vi "PingCore.vi"(8 "error in (no error)":errorcluster, 10 "Timeout (ms)":i32=60000, 11 "MicronGRPCClient in":refnum<class "MicronGRPCClient.lvclass">) -> (0 "error out":errorcluster, 2 "Response":string, 3 "MicronGRPCClient out":refnum<class "MicronGRPCClient.lvclass">)   [LabVIEW 2019, in "MicronGRPCClient.lvclass"]
uses:
  MicronGRPCClient.lvclass
  MicronCLI/Typedefs/Message.ctl
  MicronCLI/Typedefs/ServiceDetails.ctl
  MicronCLI/MicronCLI.lvclass
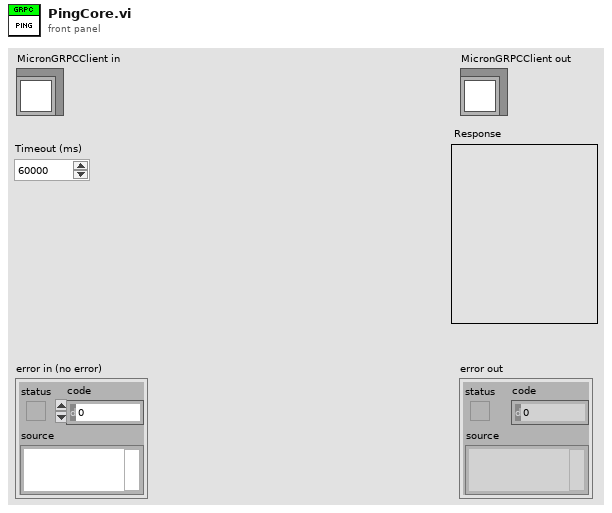
[diagram p1: front panel]
types:
  T1 = typedef "MicronCLI.lvclass/ServiceDetails.ctl" = cluster{"Network":string, "ServiceID":string}
  T2 = typedef "MicronCLI.lvclass/Message.ctl" = cluster{"Command":string, "Payload":string}
  T3 = typedef "MicronClient.lvclass/ServiceDetails.ctl" = cluster{"MicronPath":path, "Network":string, "ServiceID":string, "Port":i32, "FullyQualifiedName":string, "UI":string, "Args":string, "Mode":string, "AutoRestartOnError?":bool, "Simulate?":bool}
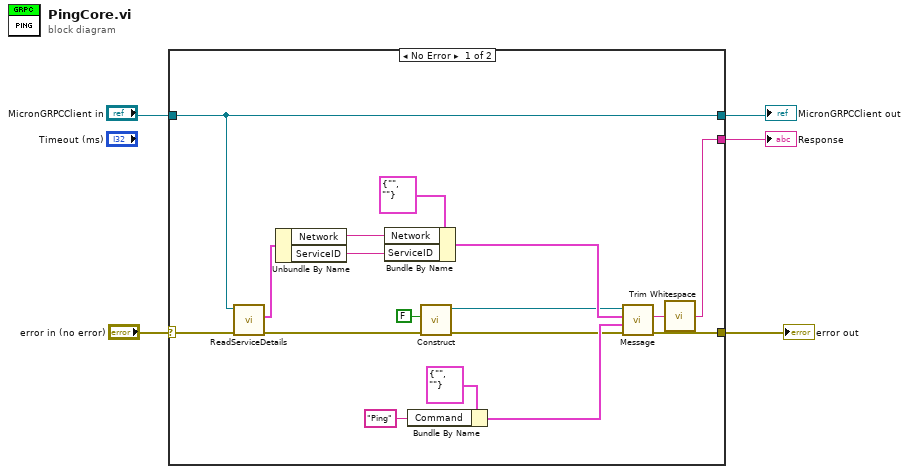
[diagram p0: block diagram]
diagram:
  n1 = case shown="No Error" "error in (no error)" {
    selector: "error in (no error)" -> [w10 w23]
    tunnel: "MicronGRPCClient in" -> [w9 w24]
    tunnel: [w6 _] -> w4
    tunnel: [w11 w23] -> w3
    tunnel: [w9 w24] -> w1
    frame No Error {
      n2 = call-dynamic "ReadServiceDetails.vi"("error in (no error)"=w10, "MicronGRPCClient in"=w9) -> ("error out"=w12:errorcluster, "ServiceDetails"=w18:T3)  [unwired: 7 in, 1 out]
      n3 = Unbundle By Name(w18) -> ("Network"=w16:string, "ServiceID"=w15:string)
      n4 = Bundle By Name(cluster=T1 {"Network"="", "ServiceID"=""} ("Service"), "Network"=w16, "ServiceID"=w15) -> (w14:T1)
      n5 = Bundle By Name(cluster=T2 {"Command"="", "Payload"=""} ("Message"), "Command"="Ping") -> (w19:T2)
      n6 = call "Construct.vi"("error in (no error)"=w12, "SkipIfNotPresent?"=FALSE) -> ("error out"=w7:errorcluster, "MicronCLI out"=w8:refnum<class "MicronCLI.lvclass">)  [unwired: 7 in, 1 out]
      n7 = call-dynamic "Message.vi"("error in (no error)"=w7, "Message"=w19, "Service"=w14, "MicronCLI in"=w8) -> ("error out"=w11:errorcluster, "Response"=w13:string)  [unwired: 5 in, 1 out]
      n8 = call <vilib>:"Trim Whitespace.vi"("string"=w13) -> ("trimmed string"=w6:string)  [unwired: 1 in]
    }
    frame Error {
    }
  }
  "error out" <- w3
  "MicronGRPCClient out" <- w1
  "Response" <- w4
